vi "Raise Internal Message.vi"(8 "Variant":variant, 9 "Internal Message Type":T1, 10 "error in (no error)":errorcluster, 11 "WAMP Client in":refnum<class "WAMP Client.lvclass">) -> (2 "error out":errorcluster, 3 "WAMP Client out":refnum<class "WAMP Client.lvclass">)   [LabVIEW 2020, in "WAMP Client.lvclass"]
uses:
  <userlib>/lvwamp/WAMP Client/WAMP Client.lvclass
  <userlib>/lvwamp/WAMP Client/WAMP Client.lvclass/WAMP Client.ctl
  <userlib>/lvwamp/WAMP Client/TypeDef/Internal Message.ctl
  <userlib>/lvwamp/WAMP Client/TypeDef/Internal Message Type.ctl
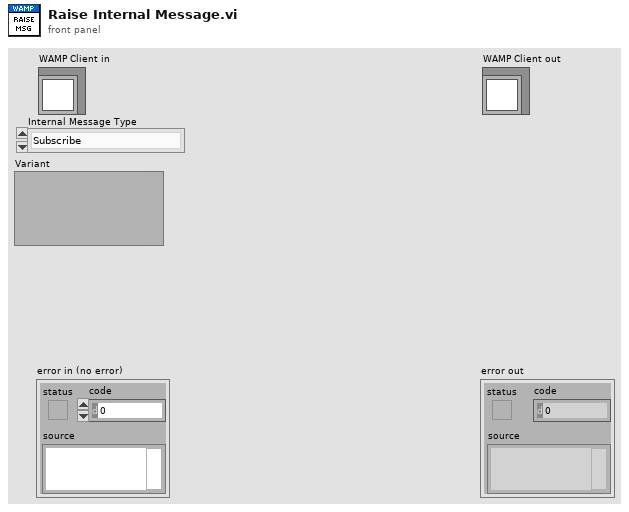
[diagram p1: front panel]
types:
  T1 = typedef "WAMP Client.lvclass/Internal Message Type.ctl" = enum16{"Subscribe", "Handle Subscribed", "Handle Event", "Unsubscribe", "Handle Unsubscribed", "Publish", "Handled Published", "Goodbye", "Handle Goodbye", "Call", "Handle Result", "Register", "Handle Registered", "Unregister", "Handle Unregistered", "Handle Invocation", "Yield"}
  T2 = typedef "WAMP Client.lvclass/Internal Message.ctl" = cluster{"Internal Message Type":T1, "Variant":variant}
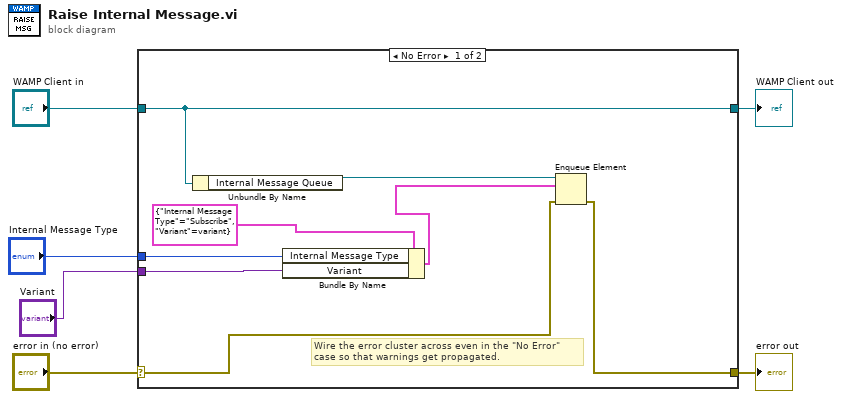
[diagram p0: block diagram]
diagram:
  n1 = case shown="No Error" "error in (no error)" {
    selector: "error in (no error)" -> [w9 w16]
    tunnel: [w10 w16] -> w5
    tunnel: [w14 w15] -> w3
    tunnel: "WAMP Client in" -> [w14 w15]
    tunnel: "Variant" -> [w12 _]
    tunnel: "Internal Message Type" -> [w7 _]
    frame No Error {
      # "Wire the error cluster across even in the \"No Error\"\ncase so that warnings get propagated."
      n2 = Unbundle By Name(w14) -> ("Internal Message Queue"=w13:refnum<queue>)
      n3 = Bundle By Name(cluster=T2 {"Internal Message Type"=enum."Subscribe", "Variant"=variant} ("Cluster"), "Internal Message Type"=w7, "Variant"=w12) -> (w11:T2)
      n4 = Enqueue Element(queue=w13, element=w11, error in (no error)=w9) -> (error out=w10:errorcluster)  [unwired: 1 in, 2 out]
    }
    frame Error {
    }
  }
  "error out" <- w5
  "WAMP Client out" <- w3
